vi "NISE.remote.Read Sys.NVMEMAreaProperties.vi"(8 "error in (no error)":errorcluster, 11 "SLSC Remote in":refnum<class "SLSC Interface.lvclass">) -> (0 "error out":errorcluster, 2 "Sys.NVMEMAreaProperties":refnum<k21>[](array[refnum]), 3 "SLSC Remote out":refnum<class "SLSC Interface.lvclass">)   [LabVIEW 2016, in "SLSC Interface.lvclass"]
uses:
  SLSC Interface Class/SLSC Interface.lvclass
  <vilib>/NI/JSON Support for LabVIEW/JSON Value/Array/Get Array Values/Get Array Values (String[]).vi
  <vilib>/NI/JSON Support for LabVIEW/JSON Value/JSON Value.lvclass
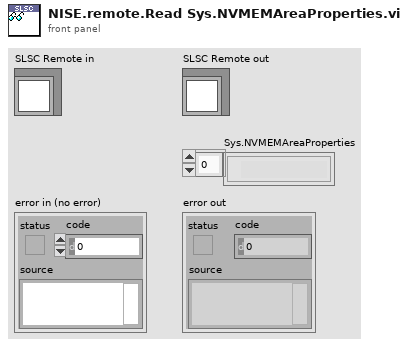
[diagram p1: front panel]
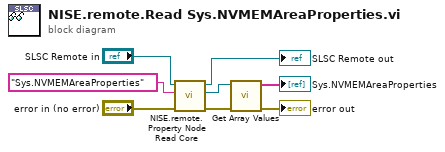
[diagram p0: block diagram]
diagram:
  n1 = call "NISE.remote.Property Node Read Core.vi"("error in (no error)"="error in (no error)", "property"="Sys.NVMEMAreaProperties", "SLSC Remote in"="SLSC Remote in") -> ("error out"=w8:errorcluster, "JSON Value out"=w3:refnum<class "JSON Value.lvclass">, "SLSC Remote out"=→"SLSC Remote out":refnum<class "SLSC Interface.lvclass">)  [unwired: 6 in]
  n2 = call-poly <vilib>:"Get Array Values.vi"("error in (no error)"=w8, "JSON Value in"=w3) -> ("error out"=→"error out":errorcluster, "values"=→"Sys.NVMEMAreaProperties":string[])  [unwired: 8 in]
